vi "MeasureDMM.vi"(8 "error in (no error)":errorcluster, 11 "Input parameters":T1={"Measurement type"=enum."Debug", "Sensor type"=enum."HPK_8in_256", "Identifier"="test.txt", "Open after execution?"=FALSE, "Plot after execution?"=FALSE, "Display channel"=0, "Voltage Delay (s)"=0.5, "Switch Delay (s)"=0.01, "VISA resource name source"="", "VISA resource name DMM"="", "VISA resource name LCR"="", "Compliance  Level (uA)"=10.0, "Voltage Limit (V)"=1000.0, "Data storage location"="", "Scan voltages"="", "Use source as DMM?"=FALSE, "LCR signal frequenzy (Hz)"=10.0, "DMM device"=enum."Keithley2001", "Sampling number"=1, "Use env. sensors on"=enum."Sensirion sht1x/7x", "Switchboard Handle"=0, "Use Switchboard"=FALSE, "LCR signal voltage (V)"=10000.0, "Repeat"=1, "Test Run Limit (nA)"=10.0, "Scan voltages IV"="", "Scan voltages CV"="", "Hex pad numbers?"=FALSE, "Set measurement type"=enum."Debug", "Custom pad scan"="", "IV voltage Delay (s)"=0.5, "CV voltage Delay (s)"=0.5} {"CV voltage Delay (s)" format="%#_13g"; "IV voltage Delay (s)" format="%#_13g"; "Voltage Limit (V)" format="%#_13g"; "Voltage Delay (s)" format="%#_13g"; "Switch Delay (s)" format="%#_13g"}) -> (0 "error out":errorcluster, 2 "Error":dbl, 3 "Result":dbl)   [LabVIEW 2016]
uses:
  Input_parameters.ctl
  instr.lib/Keithley 2450/Keithley 2450.lvlib
  instr.lib/Keithley 24XX/Keithley 24XX.lvlib
  <vilib>/Analysis/NI_AALBase.lvlib
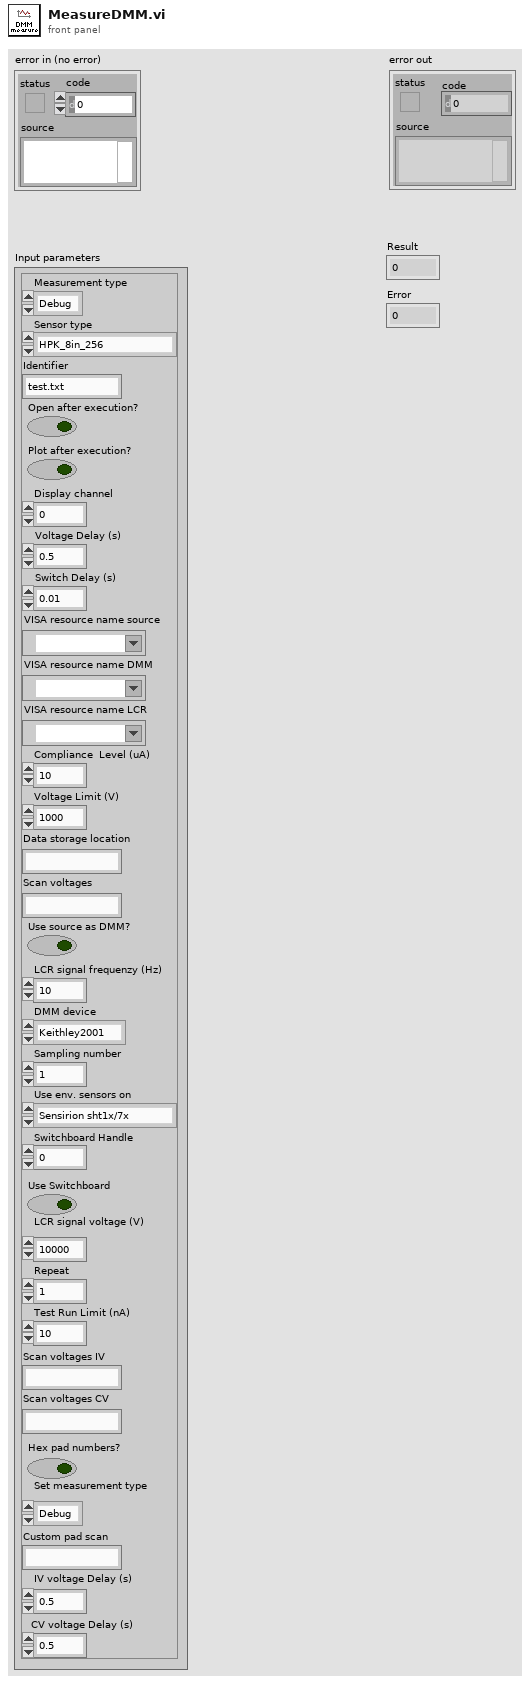
[diagram p1: front panel]
types:
  T1 = typedef "Input_parameters.ctl" = cluster{"Measurement type":enum16{"IV", "CV", "Debug", "Test"}, "Sensor type":enum16{"HPK_6in_135", "HPK_8in_256", "INF_8in_256", "Diode", "HPK_6in_256", "Test capacitances", "Full matrix"}, "Identifier":string, "Open after execution?":bool, "Plot after execution?":bool, "Display channel":i32, "Voltage Delay (s)":dbl, "Switch Delay (s)":dbl, "VISA resource name source":refnum<visa-resource-name>, "VISA resource name DMM":refnum<visa-resource-name>, "VISA resource name LCR":refnum<visa-resource-name>, "Compliance  Level (uA)":dbl, "Voltage Limit (V)":dbl, "Data storage location":string, "Scan voltages":string, "Use source as DMM?":bool, "LCR signal frequenzy (Hz)":dbl, "DMM device":enum16{"Keithley2001", "Keithley2450", "Keithley2410", "Keithley6487"}, "Sampling number":i32, "Use env. sensors on":enum16{"Sensirion sht1x/7x", "Switch Matrix", "Probecard"}, "Switchboard Handle":u32, "Use Switchboard":bool, "LCR signal voltage (V)":dbl, "Repeat":i32, "Test Run Limit (nA)":dbl, "Scan voltages IV":string, "Scan voltages CV":string, "Hex pad numbers?":bool, "Set measurement type":enum16{"IV", "CV", "Debug", "Test", "IV+CV"}, "Custom pad scan":string, "IV voltage Delay (s)":dbl, "CV voltage Delay (s)":dbl}
  T2 = enum16{"Keithley2001", "Keithley2450", "Keithley2410", "Keithley6487"}
  T3 = cluster{"error":bool, "code":i32, "source":string}
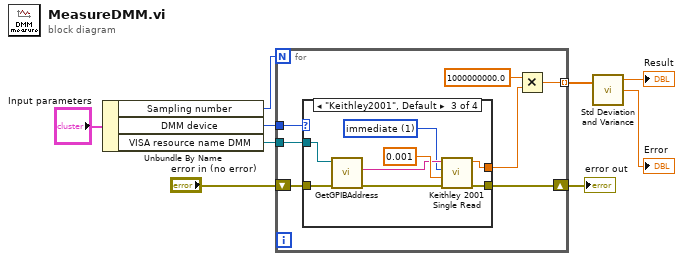
[diagram p0: block diagram]
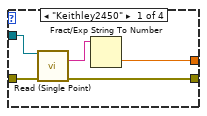
[diagram p2: hidden frame]
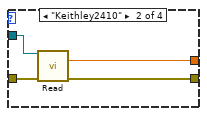
[diagram p3: hidden frame]
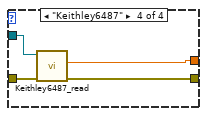
[diagram p4: hidden frame]
diagram:
  n1 = Unbundle By Name("Input parameters") -> ("Sampling number"=w4:i32, "DMM device"=w7:T2, "VISA resource name DMM"=w6:refnum<visa-resource-name>)
  n2 = for {
    N: w4 -> [_]
    tunnel: w7 -> [w15]
    tunnel: w6 -> [w14]
    tunnel: [w10] -> w3 mode=indexing
    shift-right: [w16] -> w9
    shift-left: "error in (no error)" -> [w13]
    n3 = case shown="\"Keithley2001\", Default" w15 {
      tunnel: w13 -> [w20 w25 w30 w35]
      tunnel: w14 -> [w19 w22 w27 w36]
      tunnel: [w18 w24 w33 w34] -> w16
      tunnel: [w17 w23 w31 w37] -> w11
      frame "Keithley2450" {
        n4 = call "Read (Single Point).vi"("VISA resource name"=w19, "error in (no error)"=w20) -> ("Data out"=w21:string, "error out"=w18:errorcluster)  [unwired: 11 in, 1 out]
        n5 = Fract/Exp String To Number(string=w21) -> (number=w17:dbl)  [unwired: 3 in, 1 out]
      }
      frame "Keithley2410" {
        n6 = call-poly "Read.vi"("VISA resource name"=w22, "error in (no error)"=w25) -> ("Current"=w23:sgl, "error out"=w24:errorcluster)  [unwired: 7 in, 5 out]
      }
      frame "Keithley2001", Default {
        w26 = u16 1 items=["hold", "immediate", "timer", "manual", "bus", "trigger link", "external"] ("source (imm:1)")
        n7 = call "GetGPIBAddress.vi"("error in (no error)"=w30, "VISA resource name"=w27) -> ("error out"=w29:errorcluster, "GPIB address"=w28:string)  [unwired: 7 in, 1 out]
        n8 = call "Keithley 2001 Single Read.vi"("GPIB address"=w28, "source (imm:1)"=w26, "timer value (secs)"=0.001, "error in"=w29) -> ("measurement"=w31:dbl, "error out"=w33:T3)  [unwired: 4 out]
      }
      frame "Keithley6487" {
        n9 = call "Keithley6487_read.vi"("error in (no error)"=w35, "VISA resource name"=w36) -> ("error out"=w34:errorcluster, "output"=w37:dbl)  [unwired: 7 in, 1 out]
      }
    }
    n10 = Multiply(x=1000000000.0, y=w11) -> (x*y=w10:dbl)
  }
  "error out" <- w9
  n11 = call <vilib>:"Std Deviation and Variance.vi"("X"=w3) -> ("mean"=→"Result":dbl, "standard deviation"=→"Error":dbl)  [unwired: 1 in, 1 out]
